vi "Begin.vi"(8 "error in":errorcluster) -> (0 "error out":errorcluster)   [LabVIEW 2018]
doc: "Called before other user functions, this VI is expected to open initial I/O refnums, load in file data, and do all program initialization. Notice that the <B>error out</B> terminal is simply used for data flow. Wiring it to other structures or subVIs ensures that this VI runs first."
uses:
  <vilib>/Rock Robotics/SystemInterfaces/DIO/FPGA_DIOPWMChannel.ctl
  <vilib>/Rock Robotics/WPI/SafetyOutput/WPI_SafetyOutputConfigMenu.ctl
  <vilib>/Rock Robotics/WPI/DriverStation/WPI_DriverStationRobotMode2.ctl
  <vilib>/Rock Robotics/WPI/Joystick/WPI_JoystickDeviceEnum.ctl
  <vilib>/Rock Robotics/WPI/Solenoid/WPI_SolenoidChannel.ctl
  Robot Global Data.vi
  <vilib>/Rock Robotics/Network Tables/NT Write String Array.vi
  <vilib>/Rock Robotics/WPI/RobotDrive/WPI_RobotDriveOpen4MotorWithSPARK.vi
  <vilib>/Rock Robotics/WPI/Utilities/WPI_GetSetVariantRefNum.vi
  <vilib>/Rock Robotics/WPI/Solenoid/WPI_SolenoidOpenDouble.vi
  <vilib>/Rock Robotics/WPI/MotorControl/WPI_MotorControlOpen SPARK.vi
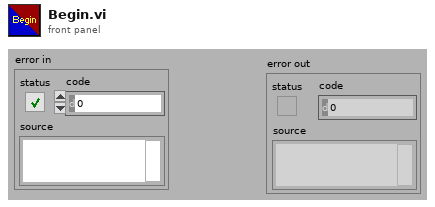
[diagram p1: front panel]
types:
  T1 = typedef "FPGA_DIOPWMChannel.ctl" = enum8{"PWM 0", "PWM 1", "PWM 2", "PWM 3", "PWM 4", "PWM 5", "PWM 6", "PWM 7", "PWM 8", "PWM 9", "PWM MXP 0", "PWM MXP 1", "PWM MXP 2", "PWM MXP 3", "PWM MXP 4", "PWM MXP 5", "PWM MXP 6", "PWM MXP 7", "PWM MXP 8", "PWM MXP 9", "Invalid"}
  T2 = typedef "WPI_SolenoidChannel.ctl" = enum8{"Solenoid 0", "Solenoid 1", "Solenoid 2", "Solenoid 3", "Solenoid 4", "Solenoid 5", "Solenoid 6", "Solenoid 7", "Invalid"}
  T3 = typedef "WPI_JoystickDeviceEnum.ctl" = enum16{"USB 0", "USB 1", "USB 2", "USB 3", "USB 4", "USB 5"}
  T4 = typedef "WPI_DriverStationRobotMode2.ctl" = enum16{"Autonomous Disabled", "Autonomous Enabled", "Teleop Disabled", "Teleop Enabled", "Disconnected", "Finish", "Test Disabled", "Test Enabled", "Emergency Stopped"}
  T5 = typedef "WPI_SafetyOutputConfigMenu.ctl" = enum16{"Enable", "Disable"}
  T6 = typedef "WPI_CompressorDevRef.ctl" = cluster{"DevStatus":errorcluster, "Pneumatics Control Module":u8}
  T7 = typedef "WPI_MotorControlDeviceRef.ctl" = cluster{"DeviceStatus":errorcluster, "Type":T8, "PWM":cluster{"PWM Channel":T1, "DeadBand":T9}, "CAN":cluster{"Device Number":u8, "SetOutput VI Ref":variant, "GetOutput VI Ref":variant, "Enable VI Ref":variant, "Disable VI Ref":variant, "Data":variant}, "Invert":bool, "DIO PWM":cluster{"PWM \"Enable\" Channel":T1, "DIOChannel":T10, "PWM Rate":dbl}}
  T8 = typedef "WPI_MotorControlType.ctl" = enum16{"PWM", "CAN", "DIO PWM"}
  T9 = typedef "WPI_PWMDeadband.ctl" = cluster{"Name":string, "maxPositivePwm":i32, "minPositivePwm":i32, "centerPwm":i32, "maxNegativePwm":i32, "minNegativePwm":i32, "angularRange":u16}
  T10 = typedef "FPGA_DIOChannel.ctl" = enum8{"DIO 0", "DIO 1", "DIO 2", "DIO 3", "DIO 4", "DIO 5", "DIO 6", "DIO 7", "DIO 8", "DIO 9", "DIO MXP 0", "DIO MXP 1", "DIO MXP 2", "DIO MXP 3", "DIO MXP 4", "DIO MXP 5", "DIO MXP 6", "DIO MXP 7", "DIO MXP 8", "DIO MXP 9", "DIO MXP 10", "DIO MXP 11", "DIO MXP 12", "DIO MXP 13", "DIO MXP 14", "DIO MXP 15", "SPI Port CS1", "SPI Port CS2", "SPI Port CS3", "SPI Port MISO", "SPI Port MOSI", "Invalid"}
  T11 = typedef "WPI_JoystickDevRef.ctl" = cluster{"Device":T3}
  T12 = typedef "WPI_SolenoidDevRef.ctl" = cluster{"DevStatus":errorcluster, "Pneumatics Control Module":u8, "Forward Solenoid Channel":T2, "Reverse Solenoid Channel":T2}
  T13 = typedef "WPI_RobotDriveDevRef.ctl" = cluster{"DevStatus":errorcluster, "Motors[]":T7[], "Square Inputs":bool, "Max Output":dbl}
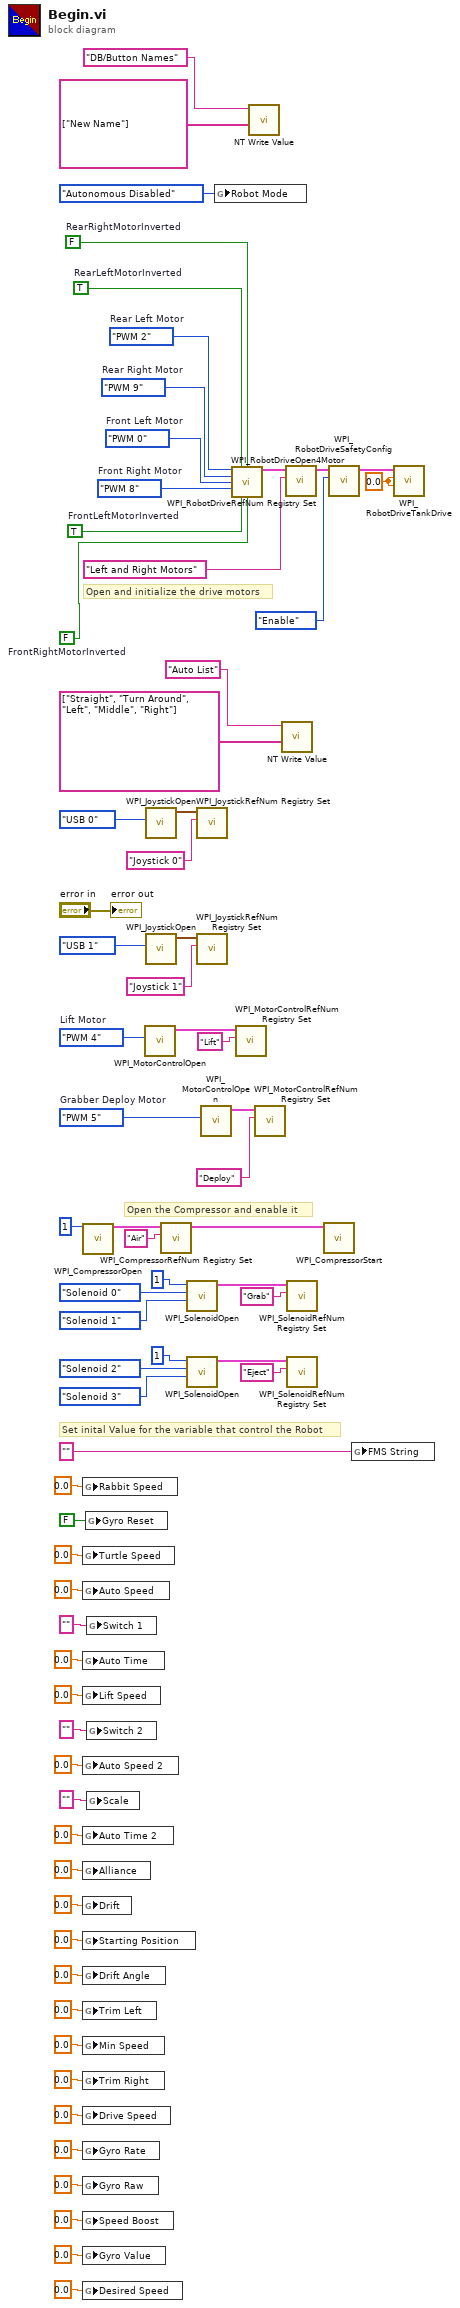
[diagram p0: block diagram]
diagram:
  w1 = FPGA_DIOPWMChannel."PWM 5"  # Grabber Deploy Motor
  w4 = FPGA_DIOPWMChannel."PWM 4"  # Lift Motor
  w16 = 0.0 ("Left axis value")
  w51 = FALSE  # FrontRightMotorInverted
  w52 = TRUE  # FrontLeftMotorInverted
  w55 = FPGA_DIOPWMChannel."PWM 8"  # Front Right Motor
  w56 = FPGA_DIOPWMChannel."PWM 0"  # Front Left Motor
  w57 = FPGA_DIOPWMChannel."PWM 9"  # Rear Right Motor
  w58 = FPGA_DIOPWMChannel."PWM 2"  # Rear Left Motor
  w53 = TRUE  # RearLeftMotorInverted
  w54 = FALSE  # RearRightMotorInverted
  # "Set inital Value for the variable that control the Robot"
  # "Open and initialize the drive motors"
  # "Open the Compressor and enable it"
  n1 = call <vilib>:"WPI_CompressorOpen.vi"("Pneumatics Control Module (0)"=u8 1) -> ("CompressorDevRef"=w47:T6)  [unwired: 13 in, 1 out]
  n2 = global write "Robot Global Data.vi" "Rabbit Speed"(0.0 ("Alliance")) -> ()
  n3 = global write "Robot Global Data.vi" "Turtle Speed"(0.0 ("Alliance")) -> ()
  n4 = global write "Robot Global Data.vi" "Auto Speed"(0.0 ("Auto Speed")) -> ()
  n5 = global write "Robot Global Data.vi" "Auto Time"(0.0 ("Auto Time")) -> ()
  n6 = global write "Robot Global Data.vi" "Lift Speed"(0.0 ("Alliance")) -> ()
  n7 = global write "Robot Global Data.vi" "Auto Speed 2"(0.0 ("Auto Speed")) -> ()
  n8 = global write "Robot Global Data.vi" "Auto Time 2"(0.0 ("Auto Time")) -> ()
  n9 = global write "Robot Global Data.vi" "Alliance"(0.0 ("Alliance")) -> ()
  n10 = global write "Robot Global Data.vi" "Drift"(0.0 ("Drift")) -> ()
  n11 = global write "Robot Global Data.vi" "Starting Position"(0.0 ("Starting Position")) -> ()
  n12 = global write "Robot Global Data.vi" "Drift Angle"(0.0 ("Drift")) -> ()
  n13 = global write "Robot Global Data.vi" "Trim Left"(0.0 ("Alliance")) -> ()
  n14 = global write "Robot Global Data.vi" "Min Speed"(0.0 ("Alliance")) -> ()
  n15 = global write "Robot Global Data.vi" "Trim Right"(0.0 ("Alliance")) -> ()
  n16 = global write "Robot Global Data.vi" "Drive Speed"(0.0 ("Alliance")) -> ()
  n17 = global write "Robot Global Data.vi" "Gyro Rate"(0.0 ("Alliance")) -> ()
  n18 = global write "Robot Global Data.vi" "Gyro Raw"(0.0 ("Alliance")) -> ()
  n19 = global write "Robot Global Data.vi" "Speed Boost"(0.0 ("Alliance")) -> ()
  n20 = global write "Robot Global Data.vi" "Gyro Value"(0.0 ("Alliance")) -> ()
  n21 = global write "Robot Global Data.vi" "Desired Speed"(0.0 ("Alliance")) -> ()
  n22 = global write "Robot Global Data.vi" "Gyro Reset"(FALSE ("Gyro Reset")) -> ()
  n23 = global write "Robot Global Data.vi" "Switch 1"("" ("Switch 1")) -> ()
  n24 = global write "Robot Global Data.vi" "Switch 2"("" ("Switch 2")) -> ()
  n25 = global write "Robot Global Data.vi" "Scale"("" ("Scale")) -> ()
  n26 = call-poly <vilib>:"WPI_MotorControlOpen.vi"("PWM Channel"=w4) -> ("MotorControlDeviceRef"=w6:T7)  [unwired: 9 in, 1 out]
  n27 = call <vilib>:"WPI_JoystickOpen.vi"("JoystickDevice"=WPI_JoystickDeviceEnum."USB 0") -> ("JoystickDevRef"=w66:T11)  [unwired: 10 in]
  n28 = call <vilib>:"WPI_JoystickOpen.vi"("JoystickDevice"=WPI_JoystickDeviceEnum."USB 1") -> ("JoystickDevRef"=w49:T11)  [unwired: 10 in]
  n29 = call <vilib>:"WPI_CompressorRefNum Registry Set.vi"("refnum name"="Air", "CompressorDevRef"=w47) -> ("CompressorDevRef"=w45:T6)  [unwired: 8 in, 1 out]
  n30 = call-poly <vilib>:"WPI_SolenoidOpen.vi"("Reverse Solenoid Channel"=WPI_SolenoidChannel."Solenoid 1", "Forward Solenoid Channel"=WPI_SolenoidChannel."Solenoid 0", "Pneumatics Control Module (0)"=u8 1) -> ("SolenoidDevRef"=w22:T12)  [unwired: 7 in, 1 out]
  n31 = call-poly <vilib>:"WPI_SolenoidOpen.vi"("Reverse Solenoid Channel"=WPI_SolenoidChannel."Solenoid 3", "Forward Solenoid Channel"=WPI_SolenoidChannel."Solenoid 2", "Pneumatics Control Module (0)"=u8 1) -> ("SolenoidDevRef"=w29:T12)  [unwired: 7 in, 1 out]
  n32 = call <vilib>:"WPI_JoystickRefNum Registry Set.vi"("refnum name"="Joystick 0", "JoystickDevRef"=w66) -> ()  [unwired: 8 in, 2 out]
  n33 = call <vilib>:"WPI_JoystickRefNum Registry Set.vi"("refnum name"="Joystick 1", "JoystickDevRef"=w49) -> ()  [unwired: 8 in, 2 out]
  n34 = call-poly <vilib>:"WPI_MotorControlOpen.vi"("PWM Channel"=w1) -> ("MotorControlDeviceRef"=w3:T7)  [unwired: 9 in, 1 out]
  n35 = global write "Robot Global Data.vi" "Robot Mode"(WPI_DriverStationRobotMode2."Autonomous Disabled" ("Robot Mode")) -> ()
  n36 = call-poly <vilib>:"WPI_RobotDriveOpen4Motor.vi"("Rear Left Motor"=w58, "Rear Left Motor Inverted"=w53, "Rear Right Motor Inverted"=w54, "Rear Right Motor"=w57, "Front Left Motor"=w56, "Front Right Motor"=w55, "Front Left Motor Inverted"=w52, "Front Right Motor Inverted"=w51) -> ("RobotDriveDevRef"=w59:T13)  [unwired: 6 in, 1 out]
  n37 = call <vilib>:"WPI_MotorControlRefNum Registry Set.vi"("refnum name"="Lift", "MotorControlDevRef"=w6) -> ()  [unwired: 8 in, 2 out]
  n38 = call-poly <vilib>:"NT Write Value.vi"("String Array"=string[] ["New Name"], "Name"="DB/Button Names") -> ()  [unwired: 9 in, 1 out]
  n39 = call <vilib>:"WPI_MotorControlRefNum Registry Set.vi"("refnum name"="Deploy", "MotorControlDevRef"=w3) -> ()  [unwired: 8 in, 2 out]
  n40 = call-poly <vilib>:"NT Write Value.vi"("String Array"=string[] ["Straight", "Turn Around", "Left", "Middle", "Right"], "Name"="Auto List") -> ()  [unwired: 9 in, 1 out]
  n41 = call <vilib>:"WPI_RobotDriveRefNum Registry Set.vi"("refnum name"="Left and Right Motors", "RobotDriveDevRef"=w59) -> ("RobotDriveDevRef"=w70:T13)  [unwired: 2 in, 7 out]
  n42 = call <vilib>:"WPI_SolenoidRefNum Registry Set.vi"("refnum name"="Grab", "SolenoidDevRef"=w22) -> ()  [unwired: 8 in, 2 out]
  n43 = call <vilib>:"WPI_SolenoidRefNum Registry Set.vi"("refnum name"="Eject", "SolenoidDevRef"=w29) -> ()  [unwired: 8 in, 2 out]
  n44 = call <vilib>:"WPI_CompressorStart.vi"("CompressorDevRef"=w45) -> ()  [unwired: 9 in, 2 out]
  n45 = call <vilib>:"WPI_RobotDriveSafetyConfig.vi"("mode"=WPI_SafetyOutputConfigMenu."Enable", "RobotDriveDevRef"=w70) -> ("RobotDriveDevRef"=w17:T13)  [unwired: 8 in, 1 out]
  n46 = global write "Robot Global Data.vi" "FMS String"("" ("FMS String")) -> ()
  n47 = call <vilib>:"WPI_RobotDriveTankDrive.vi"("Right axis value"=w16, "Left axis value"=w16, "RobotDriveDevRef"=w17) -> ()  [unwired: 6 in, 3 out]
  "error out" <- "error in"
